vi "Write fpgaClockSpeed_Hz.vi"(8 "error in (no error)":errorcluster, 10 "fpgaClockSpeed_Hz":dbl, 11 "LoopConfigInternal in":refnum<class "LoopInternalConfig.lvclass">) -> (0 "error out":errorcluster, 3 "LoopConfigInternal out":refnum<class "LoopInternalConfig.lvclass">)   [LabVIEW 2013, in "ComponentData.lvlib" / "LoopInternalConfig.lvclass"]
uses:
  <userlib>/Common/Component/common_application/RT/ComponentData/ConfigurationHandler/LoopInternalConfig/LoopInternalConfig.lvclass
  <userlib>/Common/Component/common_application/RT/ComponentData/ConfigurationHandler/LoopInternalConfig/LoopInternalConfig.lvclass/LoopInternalConfig.ctl
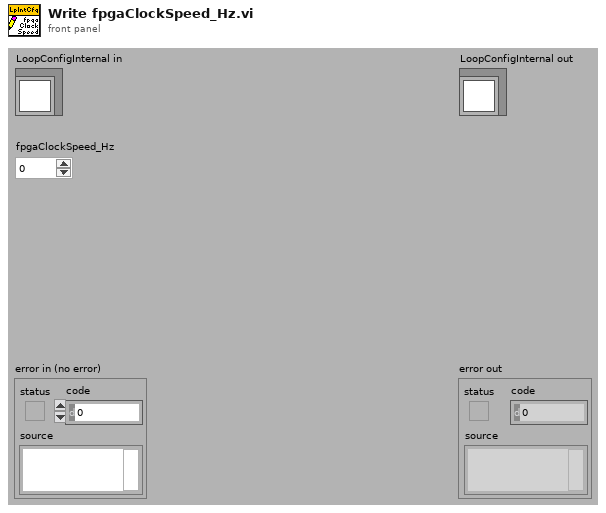
[diagram p1: front panel]
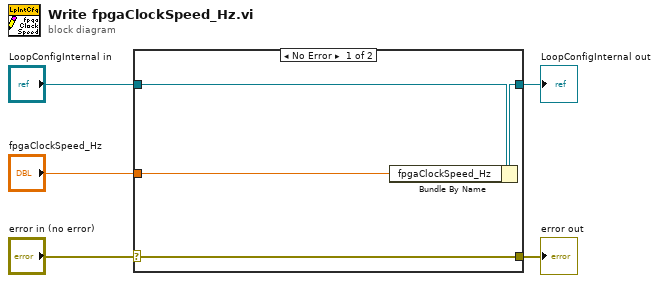
[diagram p0: block diagram]
diagram:
  n1 = case shown="No Error" "error in (no error)" {
    selector: "error in (no error)" -> [w9 w10]
    tunnel: [w9 w10] -> w4
    tunnel: [w7 w11] -> w2
    tunnel: "LoopConfigInternal in" -> [w8 w11]
    tunnel: "fpgaClockSpeed_Hz" -> [w6 _]
    frame No Error {
      n2 = Bundle By Name(cluster=w8, "fpgaClockSpeed_Hz"=w6) -> (w7:refnum<class "LoopInternalConfig.lvclass">)
    }
    frame Error {
    }
  }
  "error out" <- w4
  "LoopConfigInternal out" <- w2
